vi "Automation Update Test Name.vi"(8 "error in":errorcluster, 10 "Test Name":string, 11 "Base Software in":refnum<class "Base Software.lvclass">) -> (0 "error out":errorcluster, 3 "Base Software out":refnum<class "Base Software.lvclass">)   [LabVIEW 2019, in "Base Software.lvlib" / "Main.lvlib" / "Base Software.lvclass"]
uses:
  Project/Base Software.lvclass
  builds/Engine/Engine.lvlibp/Project/Engine.lvclass
  C:/Users/Public/Documents/Development/builds/Engine/Engine.lvlibp/Project/Engine.lvclass
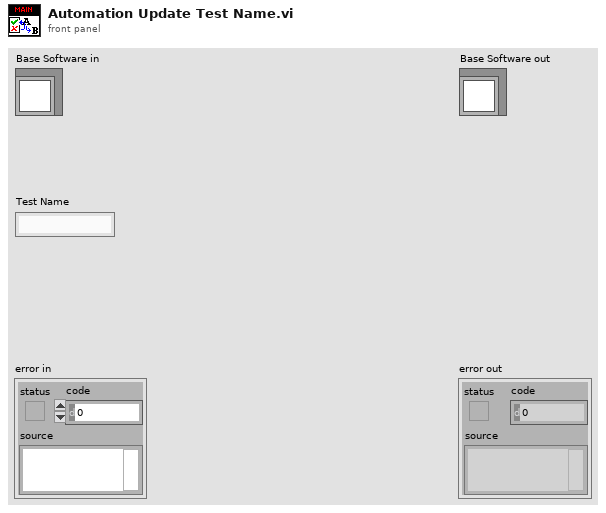
[diagram p1: front panel]
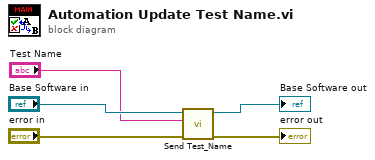
[diagram p0: block diagram]
diagram:
  n1 = call "Send Test_Name.vi"("error in"="error in", "Test Name"="Test Name", "Engine in"="Base Software in") -> ("error out"=→"error out":errorcluster, "Engine out"=→"Base Software out":refnum<class "Base Software.lvclass">)  [unwired: 7 in]
